vi "JAPCsubscribe.vi"(8 "error in (no error)":errorcluster, 11 "URL":string="VAC.VGHA_41677/PR") -> (0 "error out":errorcluster)   [LabVIEW 2014]
uses:
  Controls/DataQueue1Cluster.ctl
  Controls/DataQueue1Enum.ctl
  <userlib>/_RADE/RIO/JAPC/classes/JSubscribe/openJAPCSubscribe.vi
  <userlib>/_RADE/RIO/JAPC/classes/JSubscribe/JAPCSubscribe.vi
  <userlib>/_RADE/RIO/JAPC/classes/JSubscribe/JSubscribe.lvclass
panel:
  out "Data":variant
  out "Loop":i32
  in  "stop":bool
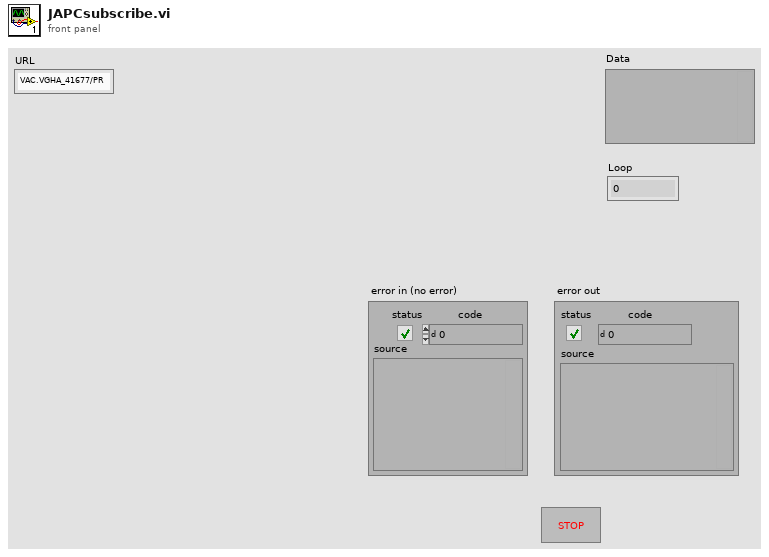
[diagram p1: front panel]
types:
  T1 = typedef "DataQueue1Cluster.ctl" = cluster{"variant":variant, "Enum":T2}
  T2 = typedef "DataQueue1Enum.ctl" = enum16{"Display", "Store"}
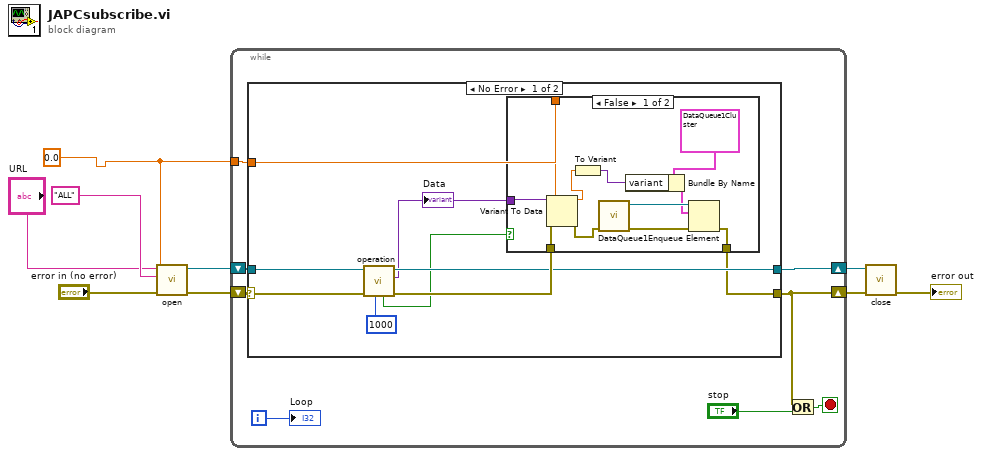
[diagram p0: block diagram]
diagram:
  w1 = 0.0
  n1 = call-poly <userlib>:"open.vi"("error in (no error)"="error in (no error)", "Data type"=w1, "Cycle"="ALL", "URL"="URL") -> ("error out"=w6:errorcluster, "Object out"=w5:refnum<class "JSubscribe.lvclass">)  [unwired: 6 in]
  n2 = while {
    shift-right: [w13] -> w4
    shift-left: w6 -> [w17]
    shift-right: [w11] -> w2
    shift-left: w5 -> [w12]
    tunnel: w1 -> [w10]
    i -> [w15]
    stop <- w14 stop-if-true
    n3 = case shown="No Error" w17 {
      selector: w17 -> [w24 w40]
      tunnel: [w18 w40] -> w13
      tunnel: w12 -> [w25 w39]
      tunnel: [w23 w39] -> w11
      tunnel: w10 -> [w22 _]
      frame No Error {
        n4 = call-poly <userlib>:"operation.vi"("Timeout (10000 ms)"=1000, "error in (no error)"=w24, "Object in"=w25) -> ("error out"=w26:errorcluster, "Data"=w21:variant, "Object out"=w23:refnum<class "JSubscribe.lvclass">, "Timeout?"=w19:bool)  [unwired: 3 in, 2 out]
        "Data" <- w21
        n5 = case shown="False" w19 {
          tunnel: w26 -> [w37 w38]
          tunnel: w21 -> [w36 _]
          tunnel: w22 -> [w35 _]
          tunnel: [w31 w38] -> w18
          frame False {
            n6 = Variant To Data(error in=w37, type=w35, Variant=w36) -> (data=w28:dbl, error out=w34:errorcluster)
            n7 = To Variant(anything=w28) -> (Variant=w29:variant)
            n8 = call "DataQueue1.vi"("error in"=w34) -> ("error out"=w33:errorcluster, "queue out"=w32:refnum<queue>)  [unwired: 8 in]
            n9 = Bundle By Name(cluster=T1 {"variant"=variant, "Enum"=enum."Store"}, "variant"=w29) -> (w27:T1)
            n10 = Enqueue Element(queue=w32, element=w27, error in (no error)=w33) -> (error out=w31:errorcluster)  [unwired: 1 in, 2 out]
          }
          frame True {
          }
        }
      }
      frame Error {
      }
    }
    n11 = Or(x=w13, y="stop") -> (x .or. y?=w14:bool)
    "Loop" <- w15
  }
  n12 = call-dynamic "close.vi"("error in (no error)"=w4, "Object in"=w2) -> ("error out"=→"error out":errorcluster)  [unwired: 9 in]
